vi "Main.vi"(8 "error in (no error)":errorcluster) -> (0 "error out":errorcluster)   [LabVIEW 2022 SP3]
uses:
  Controller/Controller/Controller.lvclass
  C:/Program Files (x86)/National Instruments/LabVIEW 2022/vi.lib/ActorFramework/Actor/Actor.lvclass
  <vilib>/ActorFramework/Report Error Msg/Report Error Msg.lvclass/Report Error Msg.ctl
  <vilib>/ActorFramework/Message Enqueuer/Message Enqueuer.lvclass/Message Enqueuer.ctl
  <vilib>/ActorFramework/Message Enqueuer/Enqueue.vi
  <vilib>/ActorFramework/Report Error Msg/Report Error Msg.lvclass
  C:/Program Files (x86)/National Instruments/LabVIEW 2022/vi.lib/ActorFramework/Message/Message.lvclass
  <vilib>/ActorFramework/Message Priority Queue/Priority Enqueue.vi
  <vilib>/ActorFramework/Actor/Actor.lvclass
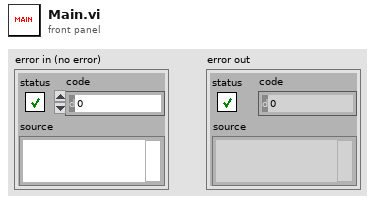
[diagram p1: front panel]
types:
  T1 = enum32{"Invalid", "Standard", "Closed", "Hidden", "Minimized", "Maximized"}
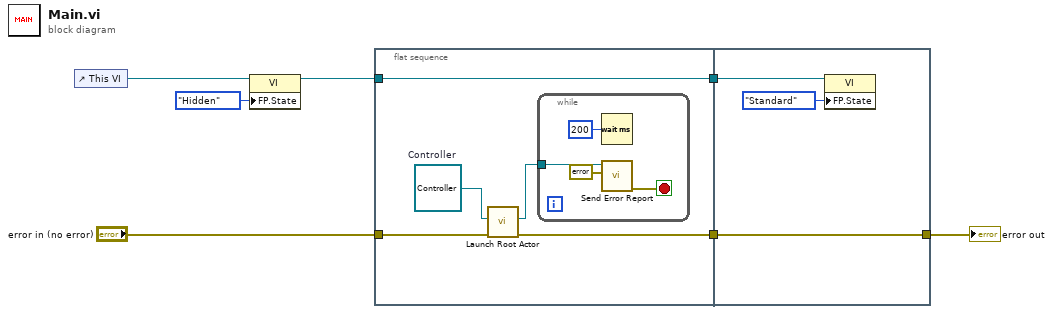
[diagram p0: block diagram]
diagram:
  n1 = control-ref of="This VI"() -> (w4:refnum<vi>)
  n2 = property class="VI"(reference=w4, "FP.State"=T1."Hidden" ("Front Panel Window:State")) -> (reference out=w2:refnum<vi>)  [unwired: 1 in, 1 out]
  n3 = flat-sequence {
    tunnel: "error in (no error)" -> [w12]
    tunnel: [w11] -> w5
    tunnel: w2 -> [w9]
    tunnel: [w9] -> w3
    tunnel: [w19] -> w6
    tunnel: w5 -> [w19]
    tunnel: w3 -> [w18]
    frame #0 {
      w10 = refnum<class "Controller.lvclass"> refnum  # Controller
      n4 = call <vilib>:"Launch Root Actor.vi"("error in (no error)"=w12, "Actor"=w10) -> ("error out"=w11:errorcluster, "Actor's Enqueuer"=w8:refnum<class "Message Enqueuer.lvclass">)  [unwired: 8 in]
      n5 = while {
        tunnel: w8 -> [w16]
        stop <- w14 stop-if-true
        n6 = Wait (ms)(milliseconds to wait=u32 200) -> ()  [unwired: 1 out]
        n7 = call <vilib>:"Send Error Report.vi"("Error From Sender"=errorcluster {"status"=FALSE, "code"=0, "source"=""}, "Message Enqueuer"=w16) -> ("error out"=w14:errorcluster)  [unwired: 9 in]
      }
    }
    frame #1 {
      n8 = property class="VI"(reference=w18, "FP.State"=T1."Standard" ("Front Panel Window:State")) -> ()  [unwired: 1 in, 2 out]
    }
  }
  "error out" <- w6
